vi "RaisedCosineFilter.vi"(6 "# of taps (1000)":u32=1000 min=1, 9 "Baud Rate":u32=9600 min=1, 10 "Roll-off Factor (0)":dbl min=0.0 max=1.0 step=0.01 format="%.2g", 11 "Signal In":waveform(dbl)) -> (3 "Signal Out":waveform(dbl))   [LabVIEW 2020]
uses:
  <vilib>/Analysis/2dsp.llb/1D Convolution (DBL).vi
  <vilib>/Analysis/NI_AALPro.lvlib
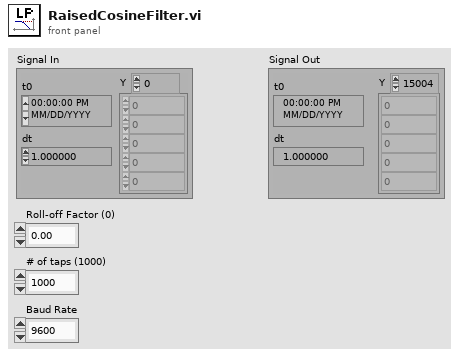
[diagram p1: front panel]
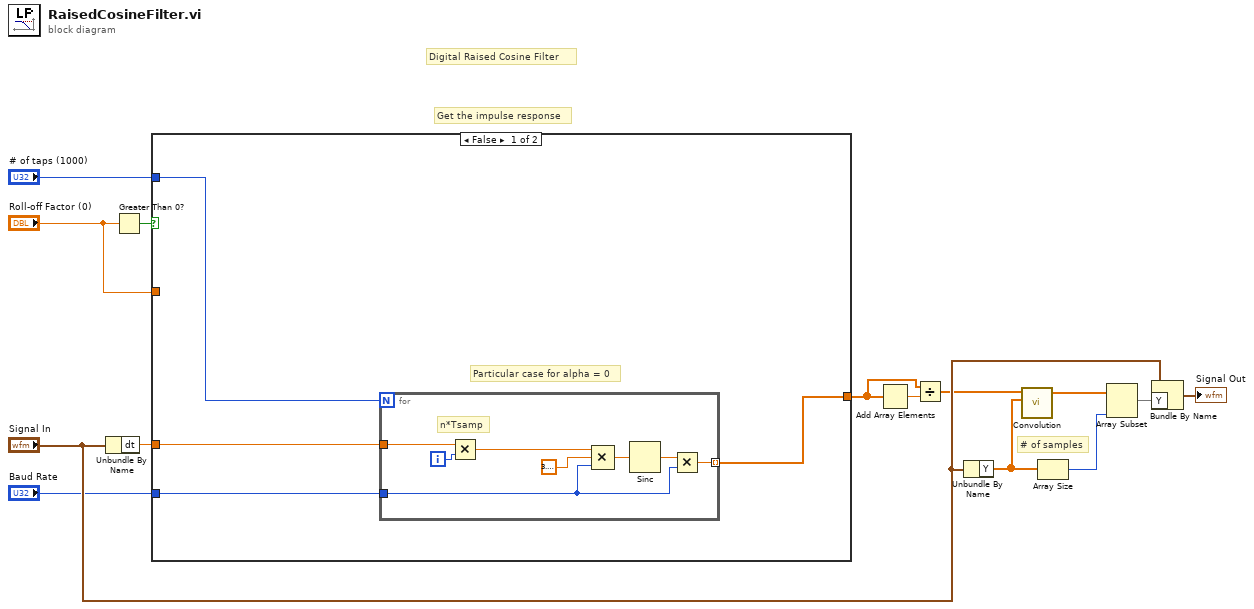
[diagram p0: block diagram]
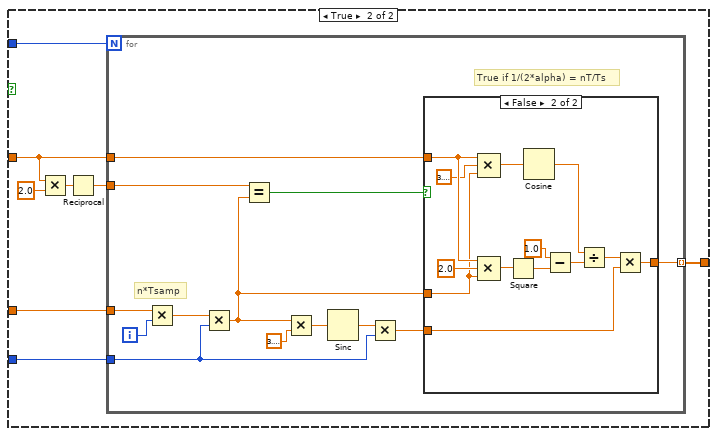
[diagram p2: hidden frame]
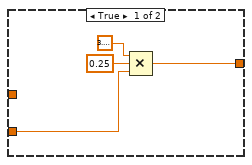
[diagram p3: hidden frame]
diagram:
  # "# of samples"
  # "Get the impulse response"
  # "Digital Raised Cosine Filter"
  n1 = Unbundle By Name("Signal In") -> ("dt"=w11:dbl)
  n2 = Greater Than 0?(x="Roll-off Factor (0)") -> (x > 0?=w14:bool)
  n3 = case shown="False" w14 {
    tunnel: "Roll-off Factor (0)" -> [_ w31]
    tunnel: "# of taps (1000)" -> [w18 w30]
    tunnel: w11 -> [w17 w29]
    tunnel: "Baud Rate" -> [w16 w28]
    tunnel: [w15 w27] -> w1
    frame False {
      # "Particular case for alpha = 0"
      n4 = for {
        N: w18 -> [_]
        tunnel: w17 -> [w25]
        tunnel: w16 -> [w20]
        tunnel: [w19] -> w15 mode=indexing
        i -> [w26]
        # "n*Tsamp"
        n5 = Multiply(x=w25, y=w26) -> (x*y=w21:dbl)
        n6 = Compound Arithmetic op=MULTIPLY(w21, 3.141592653589793, w20) -> (w22:dbl)
        n7 = Sinc(1:w22) -> (0:w23:dbl)
        n8 = Multiply(x=w23, y=w20) -> (x*y=w19:dbl)
      }
    }
    frame True {
      n9 = Multiply(x=w31, y=2.0) -> (x*y=w33:dbl)
      n10 = Reciprocal(x=w33) -> (1/x=w32:dbl)
      n11 = for {
        N: w30 -> [_]
        tunnel: w32 -> [w47]
        tunnel: w31 -> [w36]
        tunnel: [w45] -> w27 mode=indexing
        tunnel: w29 -> [w43]
        tunnel: w28 -> [w38]
        i -> [w44]
        # "True if 1/(2*alpha) = nT/Ts"
        # "n*Tsamp"
        n12 = Multiply(x=w43, y=w44) -> (x*y=w42:dbl)
        n13 = Multiply(x=w42, y=w38) -> (x*y=w35:dbl)
        n14 = Equal?(x=w47, y=w35) -> (x = y?=w46:bool)
        n15 = Multiply(x=w35, y=3.141592653589793) -> (x*y=w37:dbl)
        n16 = Sinc(1:w37) -> (0:w39:dbl)
        n17 = Multiply(x=w39, y=w38) -> (x*y=w40:dbl)
        n18 = case shown="False" w46 {
          tunnel: [w48 w57] -> w45
          tunnel: w40 -> [w49 w56]
          tunnel: w36 -> [_ w54]
          tunnel: w35 -> [_ w53]
          frame True {
            n19 = Compound Arithmetic op=MULTIPLY(3.141592653589793, 0.25 ("value"), w49) -> (w48:dbl)
          }
          frame False {
            n20 = Compound Arithmetic op=MULTIPLY(w54, 3.141592653589793, w53) -> (w55:dbl)
            n21 = Compound Arithmetic op=MULTIPLY(w54, 2.0 ("value"), w53) -> (w63:dbl)
            n22 = Square(x=w63) -> (x^2=w62:dbl)
            n23 = Cosine(x=w55) -> (cos(x)=w59:dbl)
            n24 = Subtract(x=1.0, y=w62) -> (x-y=w60:dbl)
            n25 = Divide(x=w59, y=w60) -> (x/y=w58:dbl)
            n26 = Multiply(x=w58, y=w56) -> (x*y=w57:dbl)
          }
        }
      }
    }
  }
  n27 = Add Array Elements(numeric array=w1) -> (sum=w7:dbl)
  n28 = Divide(x=w1, y=w7) -> (x/y=w6:dbl[])
  n29 = Unbundle By Name("Signal In") -> ("Y"=w3:dbl[])
  n30 = call-poly <vilib>:"Convolution.vi"("Y"=w3, "X"=w6) -> ("X * Y"=w8:dbl[])  [unwired: 8 in, 1 out]
  n31 = Array Size(array=w3) -> (size(s)=w4:i32)
  n32 = Array Subset(array=w8, length=w4) -> (w2:dbl[])  [unwired: 1 in]
  n33 = Bundle By Name(cluster="Signal In", "Y"=w2) -> (→"Signal Out":waveform(dbl))
